vi "zamien kar_obr.vi"(1 "Środek":u32[](array[numeric]), 2 "Skalowanie":u32=1 min=1, 3 "Pkt":dbl[](array[numeric])) -> (0 "pkt we wsp obrazu":cluster{i16, i16})   [LabVIEW 2016]
doc: "Zamienia ze współrzędnych kartezjańskich na współrzędne obrazu"
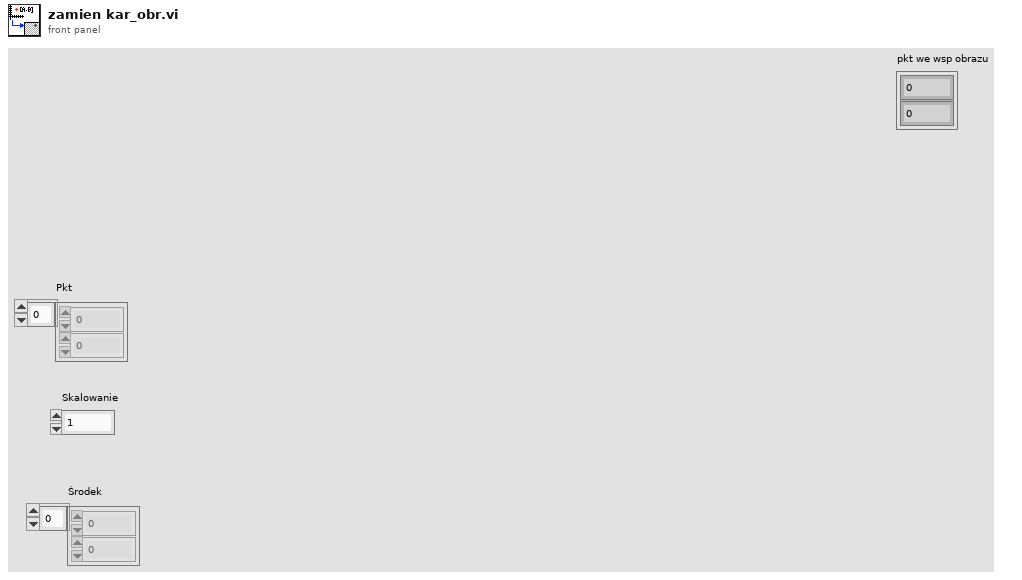
[diagram p1: front panel]
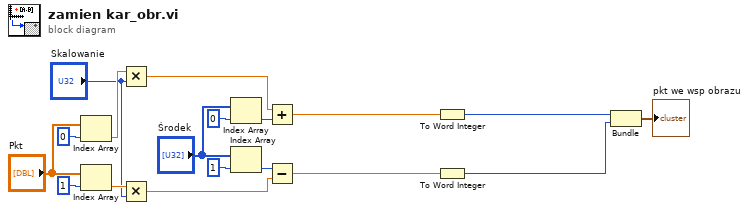
[diagram p0: block diagram]
diagram:
  n1 = Index Array(array="Pkt", index=0) -> (element=w16:dbl)
  n2 = Index Array(array="Pkt", index=1) -> (element=w14:dbl)
  n3 = Multiply(x=w16, y="Skalowanie") -> (x*y=w15:dbl)
  n4 = Multiply(x=w14, y="Skalowanie") -> (x*y=w13:dbl)
  n5 = Index Array(array="Środek", index=0) -> (element=w3:u32)
  n6 = Index Array(array="Środek", index=1) -> (element=w2:u32)
  n7 = Add(x=w15, y=w3) -> (x+y=w12:dbl)
  n8 = Subtract(x=w2, y=w13) -> (x-y=w11:dbl)
  n9 = To Word Integer(number=w12) -> (16bit integer=w8:i16)
  n10 = To Word Integer(number=w11) -> (16bit integer=w7:i16)
  n11 = Bundle(w8, w7) -> (→"pkt we wsp obrazu":cluster{i16, i16})  [unwired: 1 in]
